vi "Spring Constant.vi"() -> ()   [LabVIEW 2015]
panel:
  in  "Pressure 2":dbl
  out "Spring Constant":dbl
  out "Area":dbl
  out "Force Applied":dbl
  out "Force 2":dbl
  out "Force 1":dbl
  in  "Diameter":dbl
  in  "Pressure (psi)":dbl(knob) scale=0.0..15.0
  # "Ans b"
  # "Ans c"
  # "Ans d"
  # "Ans a"
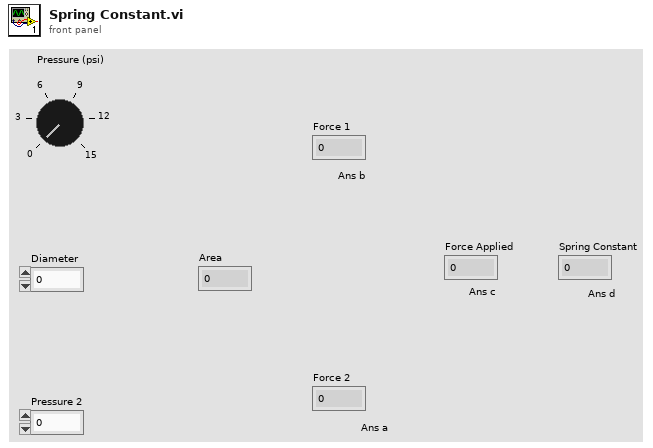
[diagram p1: front panel]
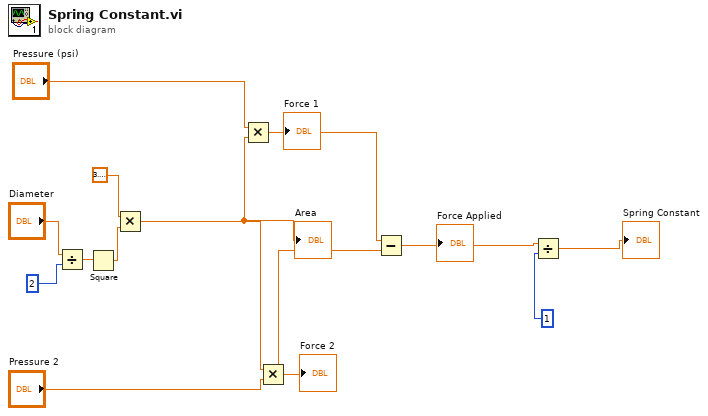
[diagram p0: block diagram]
diagram:
  n1 = Divide(x="Diameter", y=2) -> (x/y=w11:dbl)
  n2 = Square(x=w11) -> (x^2=w8:dbl)
  n3 = Multiply(x=3.141592653589793, y=w8) -> (x*y=w1:dbl)
  "Area" <- w1
  n4 = Multiply(x="Pressure (psi)", y=w1) -> (x*y=w7:dbl)
  "Force 1" <- w7
  n5 = Multiply(x=w1, y="Pressure 2") -> (x*y=w6:dbl)
  "Force 2" <- w6
  n6 = Subtract(x=w7, y=w6) -> (x-y=w5:dbl)
  "Force Applied" <- w5
  n7 = Divide(x=w5, y=1) -> (x/y=→"Spring Constant":dbl)
